vi "Configure RT AWGN.vi"(7 "Enable RT AWGN (T:Enable)":bool=TRUE, 8 "error in (no error)":errorcluster, 10 "RT AWGN Bandwidth (1 MHz)":dbl=1000000.0, 11 "VISA resource name":refnum<visa-resource-name>) -> (0 "error out":errorcluster, 3 "VISA resource name out":refnum<visa-resource-name>)   [LabVIEW 2014, in "Agilent PSG MXG Series.lvlib"]
doc: "Configures the state and flat bandwidth of real-time AWGN (additive white Gaussian noise).\n\n<B>Notes:</B>\n(1) This VI is valid only in E8267D, N5162A, N5182A, N5172B, N5182B.\n\n(2) For E8267D, this VI is valid only when the instrument installs <B>Option 403</B> (Calibrated noise, AWGN).\n\n(3) For N5162A and N5182A, this VI is valid only when the instrument installs <B>Option 651</B> or <B>Option 652</B> or <B>Option 654</B> (Internal baseband generator), and <B>Option 403</B>.\n\n(4) For N5172B and N5182B, this VI is valid only when the instrument installs <B>Option 403</B>."
uses:
  Agilent PSG MXG Series.lvlib
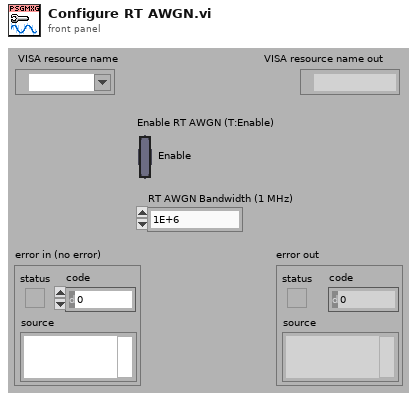
[diagram p1: front panel]
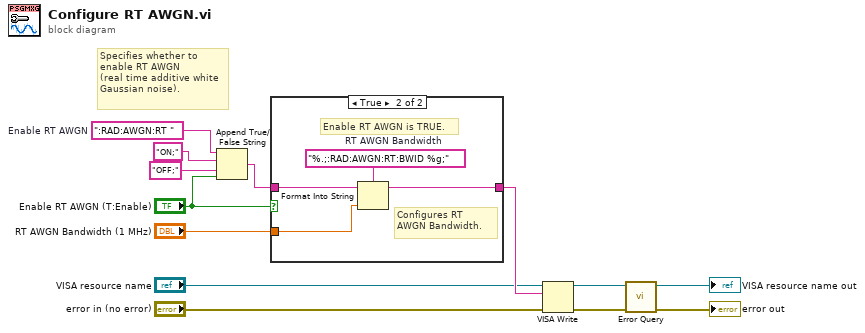
[diagram p0: block diagram]
diagram:
  w13 = ":RAD:AWGN:RT "  # Enable RT AWGN
  # "Specifies whether to\nenable RT AWGN\n(real time additive white\nGaussian noise)."
  n1 = Append True/False String(1:"Enable RT AWGN (T:Enable)", 2:"OFF;" ("false string"), 3:"ON;" ("true string"), 4:w13) -> (0:w9:string)
  n2 = case shown="True" "Enable RT AWGN (T:Enable)" {
    tunnel: w9 -> [w14 w17]
    tunnel: "RT AWGN Bandwidth (1 MHz)" -> [_ w16]
    tunnel: [w14 w15] -> w7
    frame False {
      # "Enable RT AWGN is FALSE."
    }
    frame True {
      w18 = "%.;:RAD:AWGN:RT:BWID %g;"  # RT AWGN Bandwidth
      # "Configures RT\nAWGN Bandwidth."
      # "Enable RT AWGN is TRUE."
      n3 = Format Into String(format string=w18, initial string=w17, w16) -> (resulting string=w15:string)  [unwired: 1 in, 1 out]
    }
  }
  n4 = VISA Write(VISA resource name="VISA resource name", write buffer=w7, error in (no error)="error in (no error)") -> (VISA resource name out=w6:refnum<visa-resource-name>, error out=w5:errorcluster)  [unwired: 1 out]
  n5 = call "Error Query.vi"("error in (no error)"=w5, "VISA resource name"=w6) -> ("error out"=→"error out":errorcluster, "VISA resource name out"=→"VISA resource name out":refnum<visa-resource-name>)  [unwired: 8 out]
